vi "Execute.vi"(8 "error in (no error)":errorcluster, 9 "Consumer Queues in":T1, 10 "DAC Process Command in":refnum<class "Prepare DAC Start.lvclass">, 11 "DAC Process Data in":T2) -> (0 "error out":errorcluster, 1 "Consumer Queues out":T1, 2 "Stop?":bool, 3 "DAC Process Data out":T2)   [LabVIEW 2019, in "DAC Process.lvlib" / "Prepare DAC Start.lvclass"]
uses:
  Prepare DAC Start.lvclass
  DAC Process Data.ctl
  Generic Test Stand/Generic Test Stand.lvclass
  TS Framework/ExeLogging/DAC Logger/DAC Logger.lvclass
  DAC State.ctl
  TS Framework/Consumer Queues.ctl
  UI Process/Generic UI Command/Generic UI Process Command.lvclass
  Generic DAC Command/Generic DAC Process Command.lvclass
  Trig Process/Generic Trig Command/Generic Trig Process Command.lvclass
  Generic Test Stand/Generic Test Stand.lvclass/Generic Test Stand.ctl
  UI Process/UI Acquire State/UI Acquire State.lvclass
  DAC Process.lvlib
  TS Framework/TS Framework.lvlib
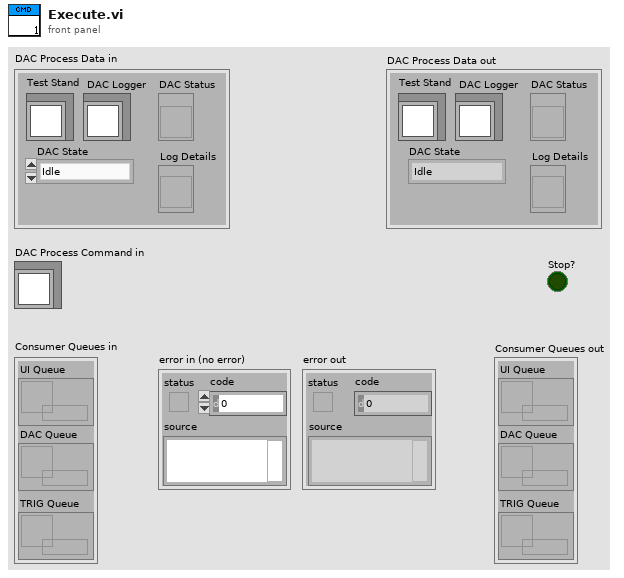
[diagram p1: front panel]
types:
  T1 = typedef "TS Framework.lvlib/Consumer Queues.ctl" = cluster{"UI Queue":refnum<queue>, "DAC Queue":refnum<queue>, "TRIG Queue":refnum<queue>}
  T2 = typedef "DAC Process.lvlib/DAC Process Data.ctl" = cluster{"Test Stand":refnum<class "Generic Test Stand.lvclass">, " DAC Logger":refnum<class "DAC Logger.lvclass">, "DAC State":T3, "DAC Status":refnum<vi>, "Log Details":refnum<vi>}
  T3 = typedef "DAC Process.lvlib/DAC State.ctl" = enum16{"Idle", "Acquiring"}
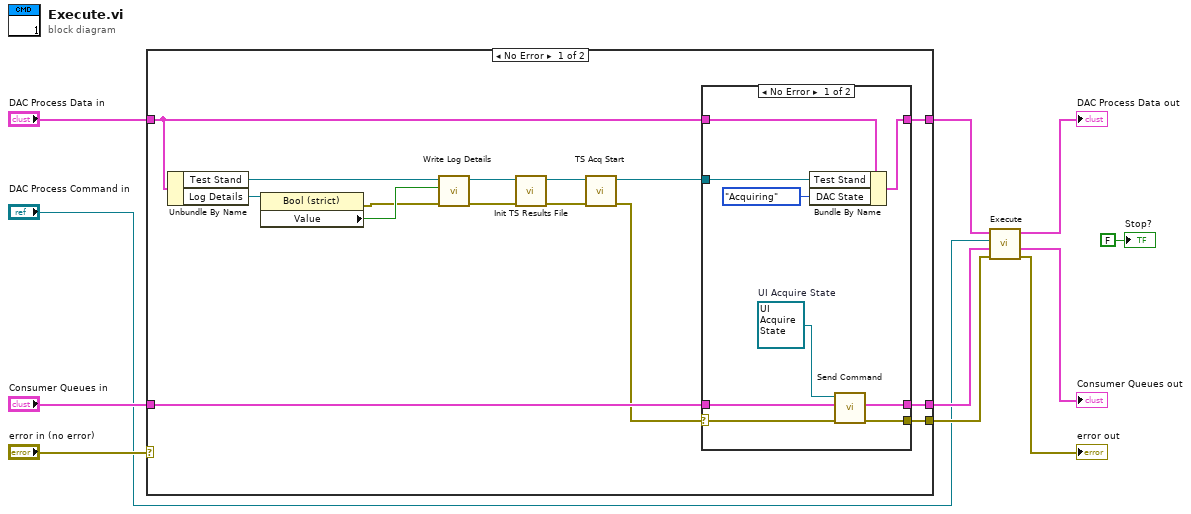
[diagram p0: block diagram]
diagram:
  n1 = case shown="No Error" "error in (no error)" {
    selector: "error in (no error)" -> [_ w41]
    tunnel: [w22 w41] -> w6
    tunnel: "Consumer Queues in" -> [w21 w40]
    tunnel: [w23 w40] -> w5
    tunnel: "DAC Process Data in" -> [w24 w39]
    tunnel: [w25 w39] -> w3
    frame No Error {
      n2 = Unbundle By Name(w24) -> ("Test Stand"=w26:refnum<class "Generic Test Stand.lvclass">, "Log Details"=w16:refnum<vi>)
      n3 = property class="Bool (strict)"(reference=w16) -> (error out=w12:errorcluster, "Value"=w13:bool)  [unwired: 1 in, 1 out]
      n4 = call "Write Log Details.vi"("error in (no error)"=w12, "Log Details"=w13, "Generic Test Stand in"=w26) -> ("error out"=w14:errorcluster, "Generic Test Stand out"=w15:refnum<class "Generic Test Stand.lvclass">)  [unwired: 7 in]
      n5 = call-dynamic "Init TS Results File.vi"("error in"=w14, "Generic Test Stand in"=w15) -> ("error out"=w19:errorcluster, "Generic Test Stand out"=w20:refnum<class "Generic Test Stand.lvclass">)  [unwired: 8 in]
      n6 = call-dynamic "TS Acq Start.vi"("error in (no error)"=w19, "Generic Test Stand in"=w20) -> ("error out"=w17:errorcluster, "Generic Test Stand out"=w18:refnum<class "Generic Test Stand.lvclass">)  [unwired: 8 in]
      n7 = case shown="No Error" w17 {
        selector: w17 -> [w27 w37]
        tunnel: w18 -> [w35 _]
        tunnel: [w33 w38] -> w25
        tunnel: w24 -> [w34 w38]
        tunnel: [w31 w36] -> w23
        tunnel: [w30 w37] -> w22
        tunnel: w21 -> [w28 w36]
        frame No Error {
          w29 = refnum<class "UI Acquire State.lvclass"> refnum  # UI Acquire State
          n8 = Bundle By Name(cluster=w34, "Test Stand"=w35, "DAC State"=DAC_State."Acquiring") -> (w33:T2)
          n9 = call-dynamic "Send Command.vi"("error in (no error)"=w27, "Consumer Queues in"=w28, "UI Process Command in"=w29) -> ("error out"=w30:errorcluster, "Consumer Queues out"=w31:T1)  [unwired: 7 in]
        }
        frame Error {
        }
      }
    }
    frame Error {
    }
  }
  n10 = call-parent "Execute.vi"("error in"=w6, "Consumer Queues in"=w5, "DAC Process Command in"="DAC Process Command in", "DAC Process Data in"=w3) -> ("error out"=→"error out":errorcluster, "Consumer Queues out"=→"Consumer Queues out":T1, "DAC Process Data out"=→"DAC Process Data out":T2)  [unwired: 4 in, 1 out]
  "Stop?" <- FALSE ("Stop?")
